vi "Init MDI.vi"(8 "error in (no error)":errorcluster caption="entrée d'erreur (pas d'erreur)", 9 "Camera monitoring container":refnum<k24>(container), 10 "Refnum VI":refnum<vi>, 11 "Container en entrée":refnum<class "Container.lvclass">) -> (0 "error out":errorcluster caption="sortie d'erreur", 1 "Container out":refnum<class "MDI Container.lvclass">, 2 "Panel Out":refnum<class "Window.lvclass">, 3 "Container en sortie":refnum<class "Container.lvclass">)   [LabVIEW 2023, in "Container.lvclass"]
uses:
  Container.lvclass
  System.Windows.Forms
  <vilib>/MGI/Panel Manager/Panel/Panel/Window/Window.lvclass
  C:/Program Files (x86)/National Instruments/LabVIEW 2023/vi.lib/MGI/Panel Manager/Panel/Panel/Panel.lvclass
  <vilib>/MGI/Panel Manager - .NET Panels/MDI/MDI Container/MDI Container.lvclass
  Container.lvclass/Container.ctl
  6c14fba2-1ba6-4e4d-bb38-0494493554c0.vi
  6c14fba2-1ba6-4e4d-bb38-0494493554c0.vi/659df739-fa42-474c-bf03-f9ba45f35773.vi
  <vilib>/MGI/Panel Manager/Panel/Window Position/Persistent Position/Persistent Position.vi
  <vilib>/MGI/Panel Manager/Panel/Panel/Window/Window.vi
  <userlib>/LV-TOML/lib/Parse TOML String.vi
  <userlib>/LV-TOML/lib/TOML to LabVIEW.vi
  <vilib>/MGI/Panel Manager/Panel/Panel.lvlib
  <vilib>/MGI/Panel Manager/Panel/Panel/Panel.lvclass
  <vilib>/MGI/Panel Manager/Panel/Window Position/Persistent Position/Persistent Position.lvclass
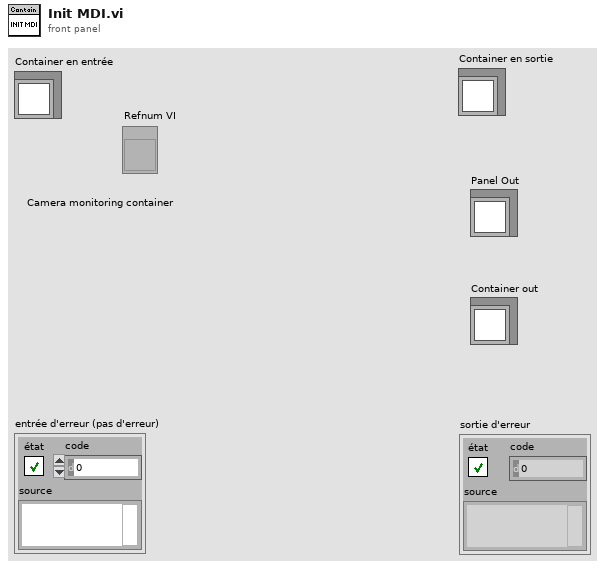
[diagram p1: front panel]
types:
  T1 = typedef "Container.lvclass/Parsed data container.ctl" = cluster{"Ctrl Config":cluster{"Caméra CP":bool, "Caméra CL":bool}}
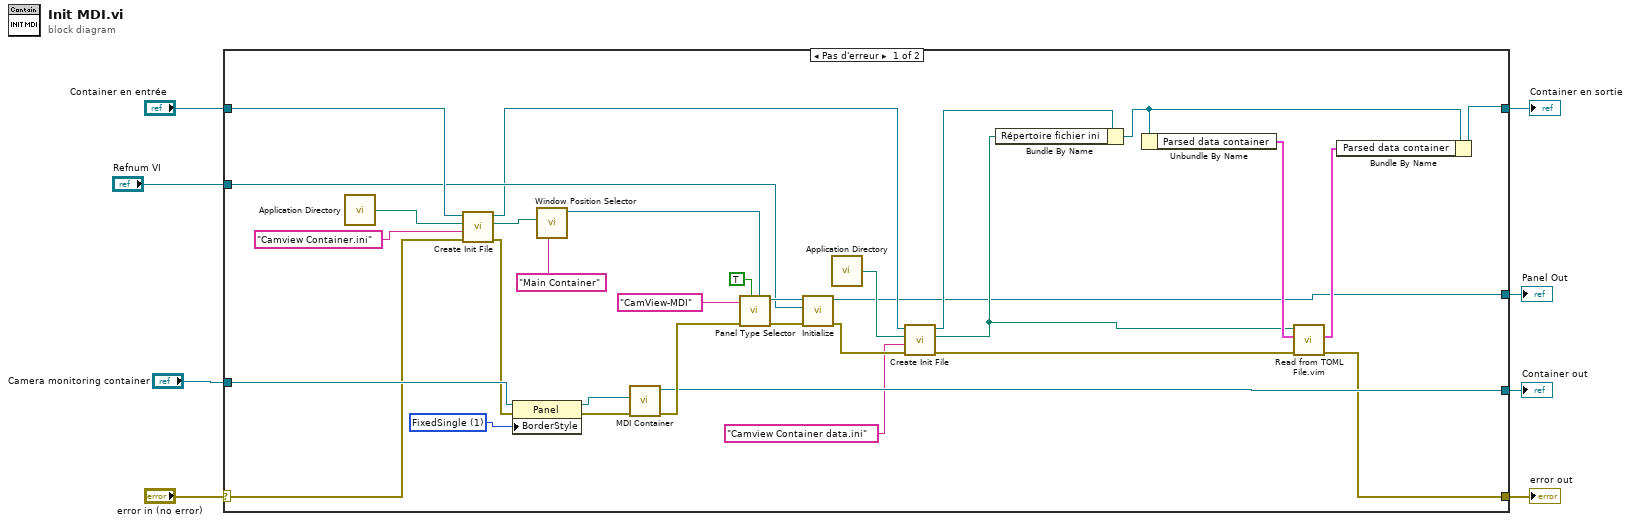
[diagram p0: block diagram]
diagram:
  n1 = case shown="Pas d'erreur" "error in (no error)" {
    selector: "error in (no error)" -> [w28 w42]
    tunnel: [w21 w42] -> w7
    tunnel: [w20 w41] -> w5
    tunnel: "Container en entrée" -> [w26 w41]
    tunnel: [w9 _] -> w4
    tunnel: [w30 _] -> w3
    tunnel: "Camera monitoring container" -> [w29 _]
    tunnel: "Refnum VI" -> [w23 _]
    frame No Error {
      w32 = 1 items=["None", "FixedSingle", "Fixed3D"] ("BorderStyle")
      n2 = call <vilib>:"Application Directory.vi"() -> ("Application Directory"=w25:path)
      n3 = call "Create Init File.vi"("error in (no error)"=w28, "Nom du fichier ini"="Camview Container.ini" ("VI ID"), "Répertoire de l'appli"=w25, "Container en entrée"=w26) -> ("error out"=w27:errorcluster, "Répertoire fichier ini out"=w22:path, "Container en sortie"=w13:refnum<class "Container.lvclass">)  [unwired: 5 in]
      n4 = property on="Nœud de propriété" class="Panel"(reference=w29, error in=w27, "BorderStyle"=w32) -> (reference out=w36:refnum<k24>, error out=w35:errorcluster)
      n5 = call-poly <vilib>:"Window Position Selector.vi"("VI ID"="Main Container", "Path"=w22) -> ("Persistent Position out"=w39:refnum<class "Window Position.lvclass">)  [unwired: 8 in, 1 out]
      n6 = call <vilib>:"MDI Container.vi"("error in (no error)"=w35, "Panel"=w36) -> ("error out"=w40:errorcluster, "Container out"=w30:refnum<class "MDI Container.lvclass">)  [unwired: 8 in]
      n7 = call-poly <vilib>:"Panel Type Selector.vi"("Window Position"=w39, "Autoshow? (T)"=TRUE, "error in (no error)"=w40, "Default Title"="CamView-MDI") -> ("error out"=w37:errorcluster, "Window out"=w38:refnum<class "Window.lvclass">)  [unwired: 6 in]
      n8 = call <vilib>:"Initialize.vi"("error in (no error)"=w37, "VI Refnum"=w23, "Panel In"=w38) -> ("error out"=w17:errorcluster, "Panel Out"=w9:refnum<class "Window.lvclass">)  [unwired: 6 in, 1 out]
      n9 = call <vilib>:"Application Directory.vi"() -> ("Application Directory"=w15:path)
      n10 = call "Create Init File.vi"("error in (no error)"=w17, "Nom du fichier ini"="Camview Container data.ini" ("VI ID"), "Répertoire de l'appli"=w15, "Container en entrée"=w13) -> ("error out"=w16:errorcluster, "Répertoire fichier ini out"=w10:path, "Container en sortie"=w12:refnum<class "Container.lvclass">)  [unwired: 5 in]
      n11 = Bundle By Name(cluster=w12, "Répertoire fichier ini"=w10) -> (w11:refnum<class "Container.lvclass">)
      n12 = Unbundle By Name(w11) -> ("Parsed data container"=w19:T1)
      n13 = call "Read from TOML File.vim"("error in (no error)"=w16, "Default Value"=w19, "file path (use dialog)"=w10) -> ("error out"=w21:errorcluster, "Value"=w18:T1)  [unwired: 6 in, 1 out]
      n14 = Bundle By Name(cluster=w11, "Parsed data container"=w18) -> (w20:refnum<class "Container.lvclass">)
    }
    frame Error {
    }
  }
  "error out" <- w7
  "Container en sortie" <- w5
  "Panel Out" <- w4
  "Container out" <- w3
